vi "Finalize To Settings.vi"(8 "error in (no error)":errorcluster, 11 "Core Threads Configuration in":refnum<class "Core Thread Configuration.lvclass">) -> (0 "error out":errorcluster, 1 "settings version":T1, 2 "settings":cluster{"key":string, "value":string}[](array[cluster]), 3 "Core Threads Configuration out":refnum<class "Core Thread Configuration.lvclass">)   [LabVIEW 2017, in "DSF Core.lvlib" / "Core Thread Configuration.lvclass"]
uses:
  Core Thread Configuration.lvclass
  Typedefs/DSF Version Info.ctl
  Core Thread Configuration.lvclass/Core Thread Configuration.ctl
  DSF Core.lvlib
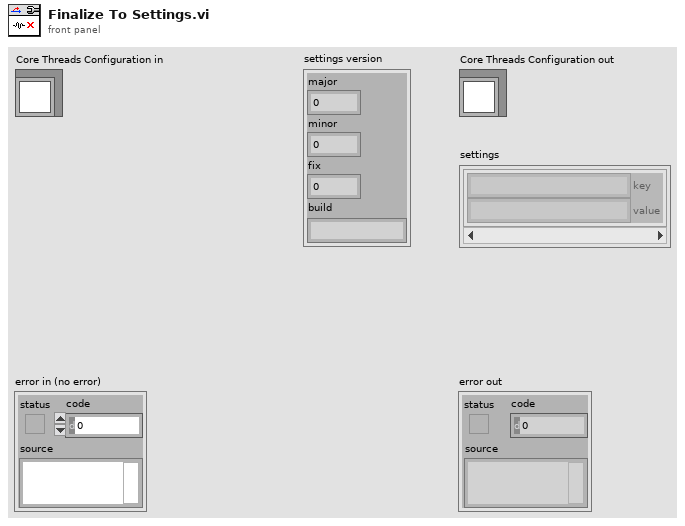
[diagram p1: front panel]
types:
  T1 = typedef "DSF Core.lvlib/DSF Version Info.ctl" = cluster{"major":u32, "minor":u32, "fix":u32, "build":string}
  T2 = typedef "DSF Core.lvlib/DSF Core Thread Configuration.ctl" = cluster{"processor":i32, "priority offset":i16}
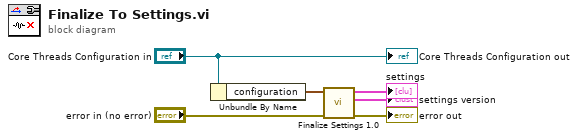
[diagram p0: block diagram]
diagram:
  n1 = Unbundle By Name("Core Threads Configuration in") -> ("configuration"=w4:T2)
  n2 = call "Finalize Settings 1.0.vi"("error in (no error)"="error in (no error)", "configuration 1.0"=w4) -> ("error out"=→"error out":errorcluster, "settings version"=→"settings version":T1, "settings 1.0"=→"settings":cluster{"key":string, "value":string}[])  [unwired: 7 in]
  "Core Threads Configuration out" <- "Core Threads Configuration in"
